vi "LfromSpaceCharge.vi"() -> ()   [LabVIEW 2018]
uses:
  <vilib>/Analysis/1siggen.llb/Ramp Pattern by Delta.vi
  <vilib>/Analysis/NI_AALBase.lvlib
panel:
  out "length when confined":dbl=0.06120041999999998
  in  "length at dump":dbl=0.079
  in  "phi at dump":dbl=4.47
  out "L*V vs L":cluster{dbl[], dbl[]}(graph)={[0.024186260000000015, 0.02662515999999998, 0.029064050000000008, 0.03147186000000002, 0.03267575, 0.034477499999999994, 0.03628745, 0.037491359999999974, 0.03869526000000001, 0.03989915999999999, 0.040497000000000005, 0.04114917000000001, 0.04239917999999998, 0.04299702999999999, 0.0436492, 0.04489921000000002, 0.04549705000000004, 0.04614921000000005, 0.04674706000000001, 0.04739922999999996, 0.047997069999999975, 0.04864923999999998, 0.04924708999999999, 0.04989926, 0.05049710000000002, 0.05049710000000002, 0.051747109999999985, 0.051747109999999985, 0.05241433000000001, 0.05301218000000002, 0.05301218000000002, 0.054277240000000004, 0.054277240000000004, 0.054277240000000004, 0.05554231000000004, 0.05554231000000004, 0.05554231000000004, 0.05680736999999997, 0.05680736999999997, 0.05680736999999997, 0.057405209999999984, 0.05807243000000001, 0.05807243000000001, 0.05807243000000001, 0.05867028000000002, 0.05933749999999999, 0.05933749999999999, 0.059935340000000004, 0.06060257000000002, 0.06060257000000002, 0.06060257000000002, 0.06120041999999998, 0.06120041999999998, 0.06186764, 0.06186764, 0.06246548000000002, 0.06246548000000002, 0.06313269999999999, 0.06313269999999999, 0.06373054, 0.06373054, 0.06434813, 0.06434813, 0.06494598000000001, 0.06494598000000001, 0.06494598000000001, 0.06556356000000002, 0.06556356000000002, 0.06616139999999998, 0.06616139999999998, 0.06677898999999998, 0.06677898999999998, 0.06677898999999998, 0.06737683, 0.06799442, 0.06799442, 0.06799442, 0.06859227000000001, 0.06859227000000001, 0.06920986000000001, 0.06920986000000001, 0.06920986000000001, 0.06980769999999997, 0.06980769999999997, 0.07042528999999997, 0.07042528999999997, 0.07042528999999997, 0.07102313999999998, 0.07164071999999999, 0.07164071999999999, 0.07164071999999999, 0.07164071999999999, 0.07164071999999999, 0.07285615000000001, 0.07285615000000001, 0.07285615000000001], [0.012093130000000007, 0.015975095999999987, 0.020344835000000006, 0.025177488000000015, 0.029408175000000005, 0.034477499999999994, 0.039916195, 0.044989631999999974, 0.05030383800000001, 0.05585882399999998, 0.06074550000000001, 0.06583867200000003, 0.07207860599999998, 0.077394654, 0.08293348, 0.08979842000000005, 0.09554380500000008, 0.10152826200000012, 0.107518238, 0.11375815199999992, 0.11999267499999994, 0.12648802399999995, 0.13296714299999998, 0.13971792800000002, 0.14644159000000007, 0.15149130000000005, 0.16041604099999995, 0.16559075199999995, 0.17296728900000005, 0.18024141200000007, 0.18554263000000007, 0.195398064, 0.20082578800000003, 0.20625351200000003, 0.21661500900000016, 0.22216924000000016, 0.22772347100000015, 0.23859095399999988, 0.2442716909999999, 0.2499524279999999, 0.25832344499999993, 0.2671331780000001, 0.27294042100000004, 0.278747664, 0.2874843720000001, 0.29668749999999994, 0.30262124999999995, 0.311663768, 0.32119362100000015, 0.32725387800000016, 0.3333141350000001, 0.3427223519999999, 0.3488423939999999, 0.35883231200000004, 0.36501907600000005, 0.3747928800000001, 0.3810394280000001, 0.39142273999999994, 0.39773601, 0.407875456, 0.41424851, 0.42469765800000003, 0.431132471, 0.4416326640000001, 0.44812726200000014, 0.4546218600000001, 0.4655012760000002, 0.47205763200000017, 0.4829782199999999, 0.4895943599999999, 0.5008424249999999, 0.5075203239999999, 0.5141982229999998, 0.525539274, 0.5371559180000001, 0.54395536, 0.550754802, 0.562456614, 0.5693158410000001, 0.5813628240000002, 0.5882838100000001, 0.5952047960000001, 0.6073269899999998, 0.6143077599999998, 0.6267850809999997, 0.6338276099999998, 0.6408701389999998, 0.653412888, 0.666258696, 0.6734227679999999, 0.6805868399999999, 0.6877509119999999, 0.694914984, 0.7139902700000001, 0.7212758850000001, 0.7285615000000001]}
  out "V vs L":cluster{dbl[], dbl[]}(graph)={[0.024186260000000015, 0.02662515999999998, 0.029064050000000008, 0.03147186000000002, 0.03267575, 0.034477499999999994, 0.03628745, 0.037491359999999974, 0.03869526000000001, 0.03989915999999999, 0.040497000000000005, 0.04114917000000001, 0.04239917999999998, 0.04299702999999999, 0.0436492, 0.04489921000000002, 0.04549705000000004, 0.04614921000000005, 0.04674706000000001, 0.04739922999999996, 0.047997069999999975, 0.04864923999999998, 0.04924708999999999, 0.04989926, 0.05049710000000002, 0.05049710000000002, 0.051747109999999985, 0.051747109999999985, 0.05241433000000001, 0.05301218000000002, 0.05301218000000002, 0.054277240000000004, 0.054277240000000004, 0.054277240000000004, 0.05554231000000004, 0.05554231000000004, 0.05554231000000004, 0.05680736999999997, 0.05680736999999997, 0.05680736999999997, 0.057405209999999984, 0.05807243000000001, 0.05807243000000001, 0.05807243000000001, 0.05867028000000002, 0.05933749999999999, 0.05933749999999999, 0.059935340000000004, 0.06060257000000002, 0.06060257000000002, 0.06060257000000002, 0.06120041999999998, 0.06120041999999998, 0.06186764, 0.06186764, 0.06246548000000002, 0.06246548000000002, 0.06313269999999999, 0.06313269999999999, 0.06373054, 0.06373054, 0.06434813, 0.06434813, 0.06494598000000001, 0.06494598000000001, 0.06494598000000001, 0.06556356000000002, 0.06556356000000002, 0.06616139999999998, 0.06616139999999998, 0.06677898999999998, 0.06677898999999998, 0.06677898999999998, 0.06737683, 0.06799442, 0.06799442, 0.06799442, 0.06859227000000001, 0.06859227000000001, 0.06920986000000001, 0.06920986000000001, 0.06920986000000001, 0.06980769999999997, 0.06980769999999997, 0.07042528999999997, 0.07042528999999997, 0.07042528999999997, 0.07102313999999998, 0.07164071999999999, 0.07164071999999999, 0.07164071999999999, 0.07164071999999999, 0.07164071999999999, 0.07285615000000001, 0.07285615000000001, 0.07285615000000001], [0.5, 0.6, 0.7, 0.8, 0.9, 1.0, 1.1, 1.2000000000000002, 1.3, 1.4, 1.5, 1.6, 1.7000000000000002, 1.8, 1.9000000000000001, 2.0, 2.1, 2.2, 2.3, 2.4000000000000004, 2.5, 2.6, 2.7, 2.8000000000000003, 2.9000000000000004, 3.0, 3.1, 3.2, 3.3000000000000003, 3.4000000000000004, 3.5, 3.6, 3.7, 3.8000000000000003, 3.9000000000000004, 4.0, 4.1, 4.2, 4.300000000000001, 4.4, 4.5, 4.6000000000000005, 4.7, 4.8, 4.9, 5.0, 5.1000000000000005, 5.2, 5.300000000000001, 5.4, 5.5, 5.6000000000000005, 5.7, 5.800000000000001, 5.9, 6.0, 6.1000000000000005, 6.2, 6.300000000000001, 6.4, 6.5, 6.6000000000000005, 6.7, 6.800000000000001, 6.9, 7.0, 7.1000000000000005, 7.2, 7.300000000000001, 7.4, 7.5, 7.6000000000000005, 7.7, 7.800000000000001, 7.9, 8.0, 8.100000000000001, 8.2, 8.3, 8.4, 8.5, 8.6, 8.700000000000001, 8.8, 8.9, 9.0, 9.1, 9.200000000000001, 9.3, 9.4, 9.5, 9.6, 9.700000000000001, 9.8, 9.9, 10.0]}
  in  "center":dbl=-0.298
  in  "delta":dbl=0.1
  in  "start":dbl=0.5
  in  "end":dbl=10.0
  in  "Fully confined":cluster{"z (mm)":dbl[], "B (T)":dbl[]}[](graph)=[{"z (mm)"=[-0.4946205487469375, -0.48862344329172347, -0.4826232674243275, -0.47662616196911345, -0.4706261041944937, -0.46462616451265015, -0.4586294133357648, -0.45263065458168356, -0.44663248629148344, -0.44063337325907354, -0.43463461450499224, -0.4286382176064356, -0.4226392226668019, -0.41664294386102146, -0.41064583840580743, -0.40464908722892207, -0.39865198177370803, -0.39265499441127016, -0.38666025081158073, -0.38066468056245767, -0.3746691103133346, -0.3686741305280926, -0.36267879646452206, -0.35668558807092354, -0.3506907263784579, -0.34469716370653064, -0.3387039553129322, -0.3327108650121099, -0.32671895563904985, -0.3207259834310039, -0.31473466452182497, -0.30874240087043636, -0.30275084577570505, -0.29675893640264506, -0.2907672632151375, -0.27932879690964096, -0.27333676944380475, -0.2673437972357587, -0.26135212404825114, -0.25535820709799534, -0.24936358159108207, -0.24336860180584013, -0.23846095282252422, -0.22755586097606212, -0.22155568510866613, -0.21555255692186442, -0.2095481297145242, -0.2035415768372119, -0.19753218973327014, -0.191521621701566, -0.18550751088657502, -0.1794919829582694, -0.1734727941539006, -0.1674510073084548, -0.1614294566485614, -0.15567689771436144, -0.14992296890395718, -0.14444164020963107, -0.13896006220833296, -0.13347473148103467, -0.12799089659556862, -0.12277913762546849, -0.11674395315455954, -0.11180517449366983, -0.1068667205879148, -0.10192920847205011, -0.0969905272377008, -0.09178035792758288, -0.08629198303094182, -0.08080810878121703, -0.07532222695429636, -0.06983831334031282, -0.06435743077425249, -0.05832855836223294, -0.05230381919738142, -0.04627778101199137, -0.04025717509430787, -0.034235860619966973, -0.028220332691661243, -0.02220456857780312, -0.01619388245332276, -0.010184022978276086, -0.004177470100963698, 0.0018263666424952474, 0.007827014880996241, 0.01382577363507742, 0.019820517234766966, 0.02581372562836548, 0.03180303696034836, 0.03779199401400268, 0.0437766997277127, 0.049760106420884354, 0.055740915072978736, 0.06171806284901016, 0.06769662773835639, 0.07312683538199505, 0.07855809273920022, 0.08371544046265322, 0.0888723158150011, 0.09429913813238788, 0.09945541252371903, 0.10460888680411173, 0.10976560863585061, 0.11464739277061287, 0.11980353004310951, 0.12522982750371303, 0.13052239801665744, 0.13581343857207862, 0.14151547741660808, 0.14748849194547142, 0.15346292358764968, 0.15943900852869497, 0.16541816388192232, 0.17139850016291192, 0.1773830877838456, 0.18336708494089837, 0.18935533343789523, 0.19534476286265445, 0.20133643605016194, 0.20733070727874647, 0.2133272222700795, 0.21932574483860823, 0.22532556642767554, 0.23132704131561, 0.23733087805906905, 0.24333483289530444, 0.24934114958706421, 0.2553479386499291, 0.2613552000838988, 0.26736387863118316, 0.2733723209929152, 0.27938229856073815, 0.2842985008351323], "B (T)"=[2.701596070156169, 2.9904155729783177, 3.076280830574092, 3.3651003333962404, 3.458771523500719, 3.5602486461139016, 3.872485946462163, 4.052022394162416, 4.270588504406199, 4.426707154580338, 4.606243602280591, 4.941898700154974, 5.105823282837809, 5.449284313220906, 5.738103816043045, 6.050341116391316, 6.339160619213455, 6.635786054544308, 7.080724207540587, 7.471020832975919, 7.86131745841125, 8.290643746390112, 8.69655223684286, 9.242967512452323, 9.680099732939889, 10.203097211023229, 10.7495124866327, 11.303733694750866, 11.936014227956102, 12.498041368582982, 13.16935156433174, 13.778214300010863, 14.433912630742212, 15.066193163947457, 15.71408556217011, 16.963034763563165, 17.587509364259688, 18.14953650488656, 18.79742890310922, 19.29700858366644, 19.749752669171432, 20.179078957150296, 20.354154871988428, 20.795747625338112, 20.881612882933887, 20.77232982781199, 20.57718151509433, 20.241526417219937, 19.718528939136597, 19.11747213596619, 18.282237357534584, 17.353331388998487, 16.182441512692503, 14.83982112119496, 13.512812594714836, 11.934453041454356, 10.26554467109289, 8.583799878383767, 6.885575894822917, 4.939296722652076, 3.0918926955915094, 1.1970025791029748, 1.0312008555073326, 2.9137966282946426, 4.774926086683013, 6.573803233314459, 8.449959111782102, 10.239772703445098, 12.387271469173715, 14.23727747373718, 16.21998433094866, 18.072592313015036, 19.724848027357936, 21.535824369377863, 23.073593073593074, 24.697227035404048, 25.96178810181452, 27.27318476327723, 28.202090731813314, 29.146608565366815, 29.755471301045937, 30.3096925091641, 30.645347607038488, 30.80146625721262, 30.74682472965167, 30.56728828195142, 30.122350128955144, 29.57593485334568, 28.771923804948898, 27.944494959025995, 26.83605254278966, 25.64174486895755, 24.275706679933894, 22.667684583140325, 21.153333676451243, 19.455977018724703, 17.828006427742224, 16.12631314084418, 14.39339612391131, 12.47226940093519, 10.69962886079134, 8.741900987607725, 6.998836258413537, 5.114093854186326, 3.332389759074035, 1.376570002725881, 0.4027489463420775, 2.2831980876894953, 4.044216461653711, 5.925446196252011, 7.7130047407458235, 9.39128023011774, 10.8666014742633, 12.263863393321781, 13.380111742066827, 14.535389753355403, 15.409654194330544, 16.205859310218614, 16.85375170844127, 17.329913591472376, 17.657762756838054, 17.852911069555716, 17.96219412467761, 17.96219412467761, 17.806075474503473, 17.642150891820634, 17.32210765896366, 16.970840696071868, 16.588350003145244, 16.112188120114148, 15.65163810210045, 15.08961096147357, 14.699314336038247]}, {"z (mm)"=array[972 elements], "B (T)"=array[972 elements]}]
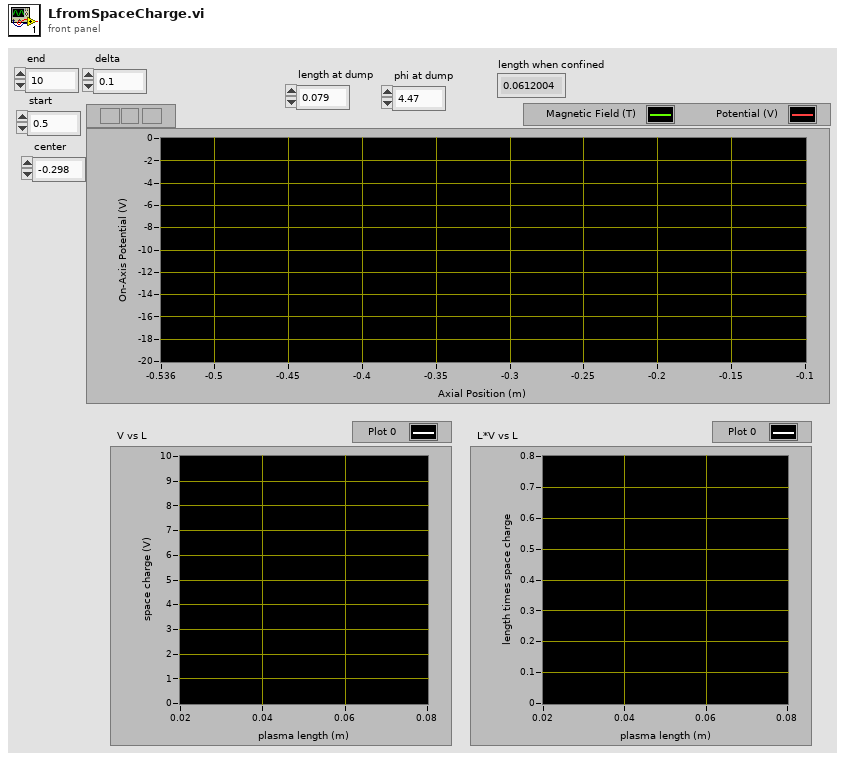
[diagram p1: front panel]
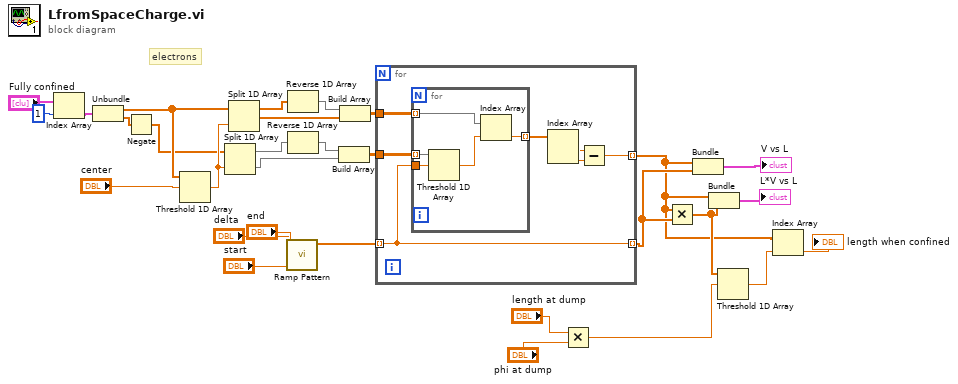
[diagram p0: block diagram]
diagram:
  # "electrons"
  n1 = Index Array(array="Fully confined", index=1) -> (element=w24:cluster{"z (mm)":dbl[], "B (T)":dbl[]})
  n2 = Unbundle(w24) -> ("z (mm)"=w23:dbl[], "B (T)"=w15:dbl[])
  n3 = Negate(x=w15) -> (-x=w14:dbl[])
  n4 = Threshold 1D Array(2:"center", 3:w23) -> (0:w20:dbl)  [unwired: 1 in]
  n5 = Split 1D Array(array=w14, index=w20) -> (first subarray=w17:dbl[], second subarray=w22:dbl[])
  n6 = Split 1D Array(array=w23, index=w20) -> (first subarray=w16:dbl[], second subarray=w21:dbl[])
  n7 = call-poly <vilib>:"Ramp Pattern.vi"("start"="start", "end"="end", "delta"="delta") -> ("Ramp Pattern"=w27:dbl[])  [unwired: 6 in, 2 out]
  n8 = Reverse 1D Array(array=w16) -> (reversed array=w2:dbl[])
  n9 = Reverse 1D Array(array=w17) -> (reversed array=w1:dbl[])
  n10 = Build Array(w1, w22) -> (w18:dbl[][])
  n11 = Build Array(w2, w21) -> (w19:dbl[][])
  n12 = for {
    tunnel: w27 -> [w31] mode=indexing
    tunnel: w19 -> [w36]
    tunnel: w18 -> [w37]
    tunnel: [w32] -> w5 mode=indexing
    tunnel: [w31] -> w13 mode=indexing
    n13 = for {
      tunnel: w37 -> [w42] mode=indexing
      tunnel: w31 -> [w41]
      tunnel: w36 -> [w38] mode=indexing
      tunnel: [w39] -> w35 mode=indexing
      n14 = Threshold 1D Array(2:w41, 3:w42) -> (0:w40:dbl)  [unwired: 1 in]
      n15 = Index Array(array=w38, index=w40) -> (element=w39:dbl)
    }
    n16 = Index Array(array=w35) -> (element #1=w34:dbl, element #2=w33:dbl)  [unwired: 2 in]
    n17 = Subtract(x=w33, y=w34) -> (x-y=w32:dbl)
  }
  n18 = Multiply(x="length at dump", y="phi at dump") -> (x*y=w6:dbl)
  n19 = Multiply(x=w5, y=w13) -> (x*y=w7:dbl[])
  n20 = Bundle(w5, w13) -> (→"V vs L":cluster{dbl[], dbl[]})  [unwired: 1 in]
  n21 = Bundle(w5, w7) -> (→"L*V vs L":cluster{dbl[], dbl[]})  [unwired: 1 in]
  n22 = Threshold 1D Array(2:w6, 3:w7) -> (0:w4:dbl)  [unwired: 1 in]
  n23 = Index Array(array=w5, index=w4) -> (element=→"length when confined":dbl)
